vi "rs3 capture single with post process.vi"(0 "frame queue in":u64, 2 "timeout":u32=5000, 3 "Processing Blocks":T4, 4 "Processing Queues":T3, 7 "error in (no error)":errorcluster, 10 "PostProcess":bool, 12 "Post-processing":T2) -> (5 "Total bocking time, ms":u32, 8 "Capture Error":string="No Error", 9 "index":i32, 13 "Processing times":T1, 14 "Frame number":u64, 15 "Time stamp":dbl, 16 "RS Format":u16(ring)=6 items=["    RS2_FORMAT_ANY             , /**< When passed to enable stream, librealsense will try to provide best suited format */", "    RS2_FORMAT_Z16             , /**< 16-bit linear depth values. The depth is meters is equal to depth scale * pixel value. */", "    RS2_FORMAT_DISPARITY16     , /**< 16-bit linear disparity values. The depth in meters is equal to depth scale / pixel value. */", "    RS2_FORMAT_XYZ32F          , /**< 32-bit floating point 3D coordinates. */", "    RS2_FORMAT_YUYV            , /**< Standard YUV pixel format as described in https://en.wikipedia.org/wiki/YUV */", "    RS2_FORMAT_RGB8            , /**< 8-bit red, green and blue channels */", "    RS2_FORMAT_BGR8            , /**< 8-bit blue, green, and red channels -- suitable for OpenCV */", "    RS2_FORMAT_RGBA8           , /**< 8-bit red, green and blue channels + constant alpha channel equal to FF */", "    RS2_FORMAT_BGRA8           , /**< 8-bit blue, green, and red channels + constant alpha channel equal to FF */", "    RS2_FORMAT_Y8              , /**< 8-bit per-pixel grayscale image */", "    RS2_FORMAT_Y16             , /**< 16-bit per-pixel grayscale image */", "    RS2_FORMAT_RAW10           , /**< Four 10-bit luminance values encoded into a 5-byte macropixel */", "    RS2_FORMAT_RAW16           , /**< 16-bit raw image */", "    RS2_FORMAT_RAW8            , /**< 8-bit raw image */", "    RS2_FORMAT_UYVY            , /**< Similar to the standard YUYV pixel format, but packed in a different order */", "    RS2_FORMAT_MOTION_RAW      , /**< Raw data from the motion sensor */", "    RS2_FORMAT_MOTION_XYZ32F   , /**< Motion data packed as 3 32-bit float values, for X, Y, and Z axis */", "    RS2_FORMAT_GPIO_RAW        , /**< Raw data from the external sensors hooked to one of the GPIO's */", "    RS2_FORMAT_COUNT             /**< Number of enumeration values. Not a valid input: intended to be used in for-loops. */"], 17 "height":i32, 20 "RS Stream":u16(ring) items=["    RS2_STREAM_ANY,", "    RS2_STREAM_DEPTH                            , /**< Native stream of depth data produced by RealSense device */", "    RS2_STREAM_COLOR                            , /**< Native stream of color data captured by RealSense device */", "    RS2_STREAM_INFRARED                         , /**< Native stream of infrared data captured by RealSense device */", "    RS2_STREAM_FISHEYE                          , /**< Native stream of fish-eye (wide) data captured from the dedicate motion camera */", "    RS2_STREAM_GYRO                             , /**< Native stream of gyroscope motion data produced by RealSense device */", "    RS2_STREAM_ACCEL                            , /**< Native stream of accelerometer motion data produced by RealSense device */", "    RS2_STREAM_GPIO                             , /**< Signals from external device connected through GPIO */", "    RS2_STREAM_COUNT"], 21 "Processed frame out":u64, 23 "error out":errorcluster, 24 "width":i32, 25 "Stream type":T6(ring), 27 "intrin post-process out":T5 {"model" items=["RS_DISTORTION_NONE", "RS_DISTORTION_MODIFIED_BROWN_CONRADY", "RS_DISTORTION_INVERSE_BROWN_CONRADY", "RS_DISTORTION_FTHETA", "RS_DISTORTION_BROWN_CONRADY", "RS_DISTORTION_COUNT"]})   [LabVIEW 2017, in "libRealSense3.lvlib"]
doc: "This VI waits for and returns the FRAME handle of captured data. (This is a BLOCKING call)\nIt also queries the frame profile to identify the type of stream data it was. \nThis type is output into the \"Stream Type\":\n\n0 Depth\n3 Color left\n5 IR Left \n9 IR Right\n21 IR Left (Y16)\n25 IR RIght (Y16) \n\nIt also starts the post-processing blocks so that temporal and spatial filters can be applied."
uses:
  libRealSense3.lvlib
panel:
  # "RS3 Capture with Post Process"
  # "(C) Intel Corp. 2018,  AGJ"
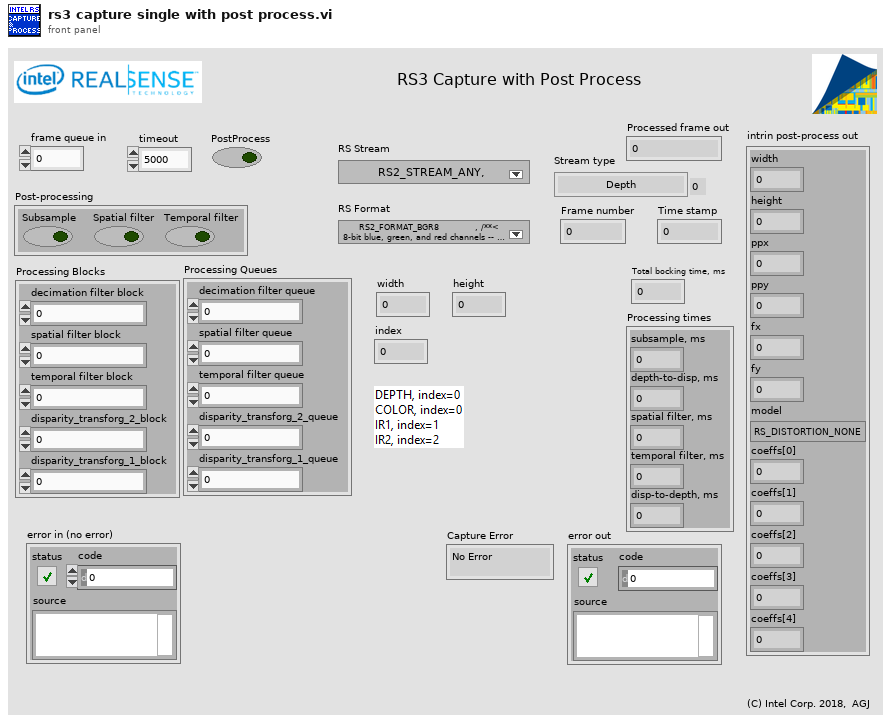
[diagram p1: front panel]
types:
  T1 = cluster{"subsample, ms":u32, "depth-to-disp, ms":u32, "spatial filter, ms":u32, "temporal filter, ms":u32, "disp-to-depth, ms":u32}
  T2 = cluster{"Subsample":bool, "Spatial filter":bool, "Temporal filter":bool}
  T3 = cluster{"decimation filter queue":u64, "spatial filter queue":u64, "temporal filter queue":u64, "disparity_transforg_2_queue":u64, "disparity_transforg_1_queue":u64}
  T4 = cluster{"decimation filter block":u64, "spatial filter block":u64, "temporal filter block":u64, "disparity_transforg_2_block":u64, "disparity_transforg_1_block":u64}
  T5 = cluster{"width":i32, "height":i32, "ppx":sgl, "ppy":sgl, "fx":sgl, "fy":sgl, "model":u32, "coeffs[0]":sgl, "coeffs[1]":sgl, "coeffs[2]":sgl, "coeffs[3]":sgl, "coeffs[4]":sgl}
  T6 = enum16{"Depth", "Color (ext.)", "Color (left) ", "IR Left", "IR Right", "IR Left (Y16)", "IR Right (Y16)"}
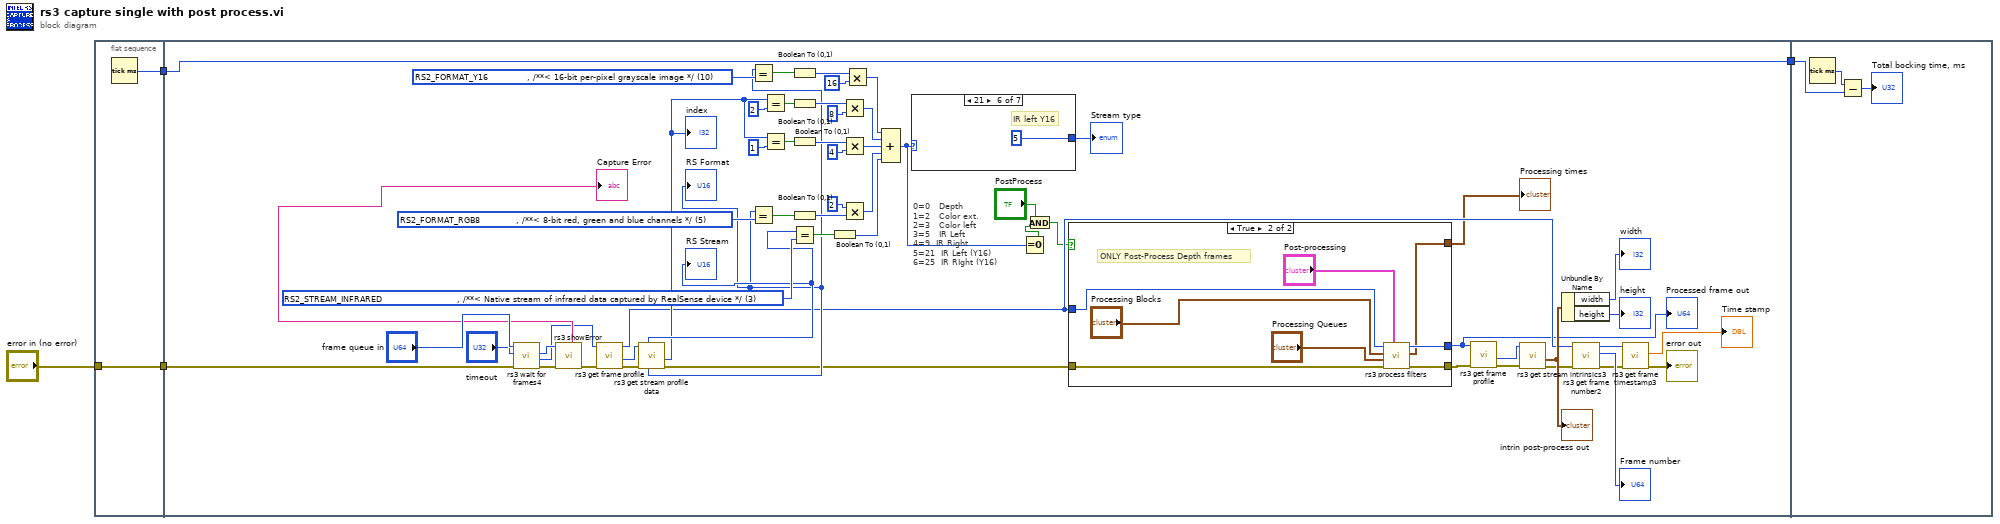
[diagram p0: block diagram]
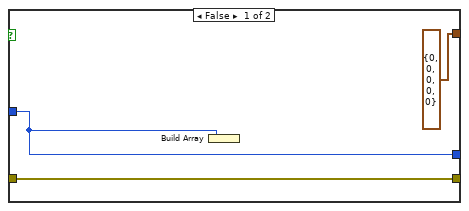
[diagram p2: hidden frame]
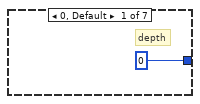
[diagram p3: hidden frame]
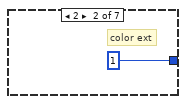
[diagram p4: hidden frame]
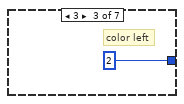
[diagram p5: hidden frame]
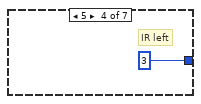
[diagram p6: hidden frame]
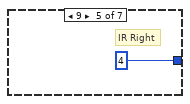
[diagram p7: hidden frame]
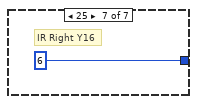
[diagram p8: hidden frame]
diagram:
  n1 = flat-sequence {
    tunnel: "error in (no error)" -> [w6]
    tunnel: [w6] -> w3
    tunnel: [w5] -> w2
    tunnel: w3 -> [w19]
    tunnel: w2 -> [w28]
    tunnel: [w28] -> w1
    tunnel: w1 -> [w84]
    frame #0 {
      n2 = Tick Count (ms)() -> (millisecond timer value=w5:u32)
    }
    frame #1 {
      w38 = u16 10 items=["    RS2_FORMAT_ANY             , /**< When passed to enable stream, librealsense will try to provide best suited format */", "    RS2_FORMAT_Z16             , /**< 16-bit linear depth values. The depth is meters is equal to depth scale * pixel value. */", "    RS2_FORMAT_DISPARITY16     , /**< 16-bit linear disparity values. The depth in meters is equal to depth scale / pixel value. */", "    RS2_FORMAT_XYZ32F          , /**< 32-bit floating point 3D coordinates. */", "    RS2_FORMAT_YUYV            , /**< Standard YUV pixel format as described in https://en.wikipedia.org/wiki/YUV */", "    RS2_FORMAT_RGB8            , /**< 8-bit red, green and blue channels */", "    RS2_FORMAT_BGR8            , /**< 8-bit blue, green, and red channels -- suitable for OpenCV */", "    RS2_FORMAT_RGBA8           , /**< 8-bit red, green and blue channels + constant alpha channel equal to FF */", "    RS2_FORMAT_BGRA8           , /**< 8-bit blue, green, and red channels + constant alpha channel equal to FF */", "    RS2_FORMAT_Y8              , /**< 8-bit per-pixel grayscale image */", "    RS2_FORMAT_Y16             , /**< 16-bit per-pixel grayscale image */", "    RS2_FORMAT_RAW10           , /**< Four 10-bit luminance values encoded into a 5-byte macropixel */", "    RS2_FORMAT_RAW16           , /**< 16-bit raw image */", "    RS2_FORMAT_RAW8            , /**< 8-bit raw image */", "    RS2_FORMAT_UYVY            , /**< Similar to the standard YUYV pixel format, but packed in a different order */", "    RS2_FORMAT_MOTION_RAW      , /**< Raw data from the motion sensor */", "    RS2_FORMAT_MOTION_XYZ32F   , /**< Motion data packed as 3 32-bit float values, for X, Y, and Z axis */", "    RS2_FORMAT_GPIO_RAW        , /**< Raw data from the external sensors hooked to one of the GPIO's */", "    RS2_FORMAT_COUNT             /**< Number of enumeration values. Not a valid input: intended to be used in for-loops. */"] ("RS Format")
      w60 = u16 3 items=["    RS2_STREAM_ANY,", "    RS2_STREAM_DEPTH                            , /**< Native stream of depth data produced by RealSense device */", "    RS2_STREAM_COLOR                            , /**< Native stream of color data captured by RealSense device */", "    RS2_STREAM_INFRARED                         , /**< Native stream of infrared data captured by RealSense device */", "    RS2_STREAM_FISHEYE                          , /**< Native stream of fish-eye (wide) data captured from the dedicate motion camera */", "    RS2_STREAM_GYRO                             , /**< Native stream of gyroscope motion data produced by RealSense device */", "    RS2_STREAM_ACCEL                            , /**< Native stream of accelerometer motion data produced by RealSense device */", "    RS2_STREAM_GPIO                             , /**< Signals from external device connected through GPIO */", "    RS2_STREAM_COUNT"] ("RS Stream")
      w37 = u16 5 items=["    RS2_FORMAT_ANY             , /**< When passed to enable stream, librealsense will try to provide best suited format */", "    RS2_FORMAT_Z16             , /**< 16-bit linear depth values. The depth is meters is equal to depth scale * pixel value. */", "    RS2_FORMAT_DISPARITY16     , /**< 16-bit linear disparity values. The depth in meters is equal to depth scale / pixel value. */", "    RS2_FORMAT_XYZ32F          , /**< 32-bit floating point 3D coordinates. */", "    RS2_FORMAT_YUYV            , /**< Standard YUV pixel format as described in https://en.wikipedia.org/wiki/YUV */", "    RS2_FORMAT_RGB8            , /**< 8-bit red, green and blue channels */", "    RS2_FORMAT_BGR8            , /**< 8-bit blue, green, and red channels -- suitable for OpenCV */", "    RS2_FORMAT_RGBA8           , /**< 8-bit red, green and blue channels + constant alpha channel equal to FF */", "    RS2_FORMAT_BGRA8           , /**< 8-bit blue, green, and red channels + constant alpha channel equal to FF */", "    RS2_FORMAT_Y8              , /**< 8-bit per-pixel grayscale image */", "    RS2_FORMAT_Y16             , /**< 16-bit per-pixel grayscale image */", "    RS2_FORMAT_RAW10           , /**< Four 10-bit luminance values encoded into a 5-byte macropixel */", "    RS2_FORMAT_RAW16           , /**< 16-bit raw image */", "    RS2_FORMAT_RAW8            , /**< 8-bit raw image */", "    RS2_FORMAT_UYVY            , /**< Similar to the standard YUYV pixel format, but packed in a different order */", "    RS2_FORMAT_MOTION_RAW      , /**< Raw data from the motion sensor */", "    RS2_FORMAT_MOTION_XYZ32F   , /**< Motion data packed as 3 32-bit float values, for X, Y, and Z axis */", "    RS2_FORMAT_GPIO_RAW        , /**< Raw data from the external sensors hooked to one of the GPIO's */", "    RS2_FORMAT_COUNT             /**< Number of enumeration values. Not a valid input: intended to be used in for-loops. */"] ("RS Format")
      # "0=0   Depth\n1=2   Color ext.\n2=3   Color left\n3=5   IR Left \n4=9  IR Right\n5=21  IR Left (Y16)\n6=25  IR RIght (Y16)"
      n3 = call "rs3 wait for frames4.vi"("error in (no error)"=w19, "timeout"="timeout", "Queue in"="frame queue in") -> (0:"error out"=w29:errorcluster, "frame"=w8:u64, 2:"error out"=w63:u64)  [unwired: 5 in, 1 out]
      n4 = call "rs3 showError.vi"("error in (no error)"=w29, "error"=w63) -> ("error out"=w23:errorcluster, "Error summary"=→"Capture Error":string)  [unwired: 5 in, 3 out]
      n5 = call "rs3 get frame profile.vi"("error in (no error)"=w23, "Frame"=w8) -> ("error out"=w22:errorcluster, "stream profile"=w27:u64, "frame out"=w17:u64)  [unwired: 6 in, 1 out]
      n6 = call "rs3 get stream profile data.vi"("error in (no error)"=w22, "Profile"=w27) -> ("error out"=w18:errorcluster, "index"=w43:i32, "RS Format"=w35:u16, "RS Stream"=w59:u16)  [unwired: 2 in, 4 out]
      "RS Format" <- w35
      "RS Stream" <- w59
      "index" <- w43
      n7 = Equal?(x=w35, y=w38) -> (x = y?=w39:bool)
      n8 = Equal?(x=w35, y=w37) -> (x = y?=w56:bool)
      n9 = Equal?(x=w43, y=2) -> (x = y?=w45:bool)
      n10 = Equal?(x=w43, y=1) -> (x = y?=w57:bool)
      n11 = Boolean To (0,1)(Boolean=w39) -> (0, 1=w41:i16)
      n12 = Boolean To (0,1)(Boolean=w45) -> (0, 1=w46:i16)
      n13 = Boolean To (0,1)(Boolean=w57) -> (0, 1=w52:i16)
      n14 = Boolean To (0,1)(Boolean=w56) -> (0, 1=w54:i16)
      n15 = Equal?(x=w59, y=w60) -> (x = y?=w55:bool)
      n16 = Boolean To (0,1)(Boolean=w55) -> (0, 1=w49:i16)
      n17 = Multiply(x=w46, y=i16 8) -> (x*y=w42:i16)
      n18 = Multiply(x=w52, y=i16 4) -> (x*y=w48:i16)
      n19 = Multiply(x=i16 2, y=w54) -> (x*y=w50:i16)
      n20 = Multiply(x=w41, y=i16 16) -> (x*y=w36:i16)
      n21 = Compound Arithmetic op=ADD(w36, w42, w48, w50, w49) -> (w16:i16)
      n22 = case shown="21" w16 {
        tunnel: [0 1 2 3 4 5 6] -> w30
        frame 0, Default {
          # "depth"
        }
        frame 2 {
          # "color ext"
        }
        frame 3 {
          # "color left"
        }
        frame 5 {
          # "IR left"
        }
        frame 9 {
          # "IR Right"
        }
        frame 21 {
          # "IR left Y16"
        }
        frame 25 {
          # "IR Right Y16"
        }
      }
      "Stream type" <- w30
      n23 = Equal To 0?(x=w16) -> (x = 0?=w14:bool)
      n24 = And(x="PostProcess", y=w14) -> (x .and. y?=w12:bool)
      n25 = case shown="True" w12 {
        tunnel: w18 -> [w67 w75]
        tunnel: [w67 w74] -> w11
        tunnel: w17 -> [w65 w73]
        tunnel: [w65 w72] -> w7
        tunnel: [T1 {"subsample, ms"=0, "depth-to-disp, ms"=0, "spatial filter, ms"=0, "temporal filter, ms"=0, "disp-to-depth, ms"=0} ("Processing times") w70] -> w15
        frame False {
          n26 = Build Array(w65) -> ()  [unwired: 1 out]
        }
        frame True {
          # "ONLY Post-Process Depth frames"
          n27 = call "rs3 process filters.vi"("Post-processing"="Post-processing", "error in (no error)"=w75, "Processing Queues"="Processing Queues", "Processing Blocks"="Processing Blocks", "Frame"=w73) -> ("error out"=w74:errorcluster, "Processing times"=w70:T1, "processed frame"=w72:u64)  [unwired: 4 in]
        }
      }
      "Processed frame out" <- w7
      "Processing times" <- w15
      n28 = call "rs3 get frame profile.vi"("error in (no error)"=w11, "Frame"=w7) -> ("error out"=w10:errorcluster, "stream profile"=w9:u64)  [unwired: 6 in, 2 out]
      n29 = call "rs3 get stream intrinsics3.vi"("error in (no error)"=w10, "stream profile"=w9) -> ("error out"=w21:errorcluster, "intrin out"=w26:T5)  [unwired: 6 in, 2 out]
      "intrin post-process out" <- w26
      n30 = Unbundle By Name(w26) -> ("width"=→"width":i32, "height"=→"height":i32)
      n31 = call "rs3 get frame number2.vi"("error in (no error)"=w21, "frame in"=w17) -> ("error out"=w31:errorcluster, "Frame number"=→"Frame number":u64, "frame out"=w34:u64)  [unwired: 6 in, 1 out]
      n32 = call "rs3 get frame timestamp3.vi"("error in (no error)"=w31, "frame in"=w34) -> ("error out"=→"error out":errorcluster, "Time stamp"=→"Time stamp":dbl)  [unwired: 6 in, 2 out]
    }
    frame #2 {
      n33 = Tick Count (ms)() -> (millisecond timer value=w85:u32)
      n34 = Subtract(x=w85, y=w84) -> (x-y=→"Total bocking time, ms":u32)
    }
  }
